vi "Offset Inline Buffers.vi"(8 "error in (no error)":errorcluster, 11 "Framework in":refnum<class "Framework.lvclass">) -> (0 "error out":errorcluster, 3 "Framework out":refnum<class "Framework.lvclass">)   [LabVIEW 2017, in "DSF Core.lvlib" / "Framework.lvclass"]
uses:
  Framework.lvclass
  Framework.lvclass/Framework.ctl
  Plugin/Plugin.lvclass
  Buffers/Buffers.lvclass
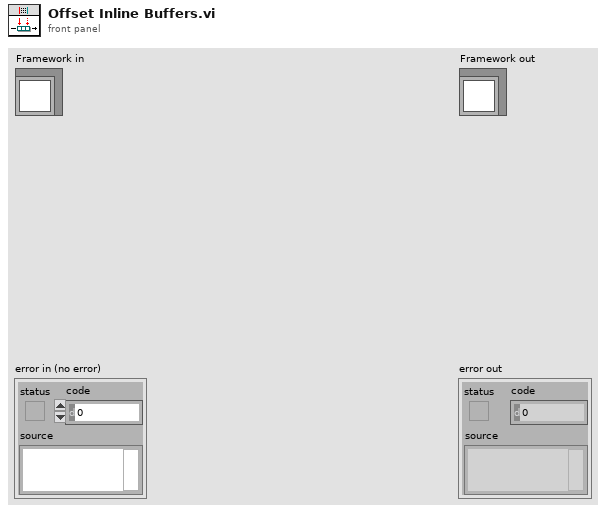
[diagram p1: front panel]
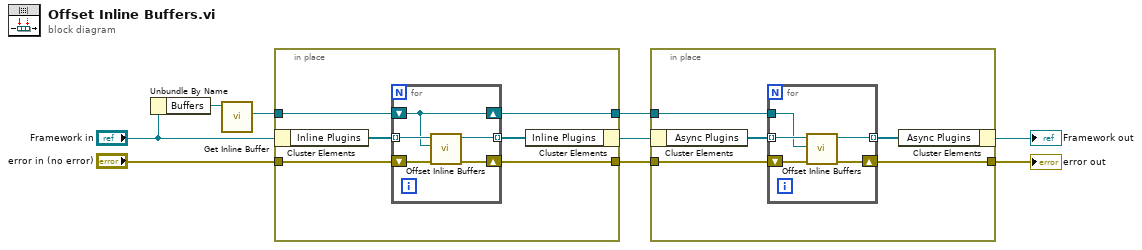
[diagram p0: block diagram]
diagram:
  n1 = Unbundle By Name("Framework in") -> ("Buffers"=w5:refnum<class "Buffers.lvclass">)
  n2 = call "Get Inline Buffer.vi"("Buffers in"=w5) -> ("Inline Buffer"=w1:refnum<class "Buffer.lvclass">)  [unwired: 9 in, 1 out]
  n3 = in-place {
    in-place-border: "error in (no error)" -> [w12]
    in-place-border: [w13] -> w8
    in-place-border: w1 -> [w11]
    in-place-border: [w10] -> w2
    n4 = in-place-cluster #1("Framework in") -> ("Inline Plugins"=w15:refnum<class "Plugin.lvclass">[])
    n5 = for {
      tunnel: w15 -> [w20] mode=indexing
      tunnel: [w19] -> w14 mode=indexing
      shift-right: [w18] -> w13
      shift-left: w12 -> [w17]
      shift-right: [w16] -> w10
      shift-left: w11 -> [w16]
      n6 = call "Offset Inline Buffers.vi"("error in (no error)"=w17, "Framework Inline Buffer"=w16, "Plugin in"=w20) -> ("error out"=w18:errorcluster, "Plugin out"=w19:refnum<class "Plugin.lvclass">)  [unwired: 7 in]
    }
    n7 = in-place-cluster #1("Inline Plugins"=w14) -> (w3:refnum<class "Framework.lvclass">)
  }
  n8 = in-place {
    in-place-border: w8 -> [w22]
    in-place-border: [w23] -> w6
    in-place-border: w2 -> [w21]
    n9 = in-place-cluster #2(w3) -> ("Async Plugins"=w25:refnum<class "Plugin.lvclass">[])
    n10 = for {
      tunnel: w25 -> [w30] mode=indexing
      tunnel: [w29] -> w24 mode=indexing
      shift-right: [w28] -> w23
      shift-left: w22 -> [w27]
      tunnel: w21 -> [w26]
      n11 = call "Offset Inline Buffers.vi"("error in (no error)"=w27, "Framework Inline Buffer"=w26, "Plugin in"=w30) -> ("error out"=w28:errorcluster, "Plugin out"=w29:refnum<class "Plugin.lvclass">)  [unwired: 7 in]
    }
    n12 = in-place-cluster #2("Async Plugins"=w24) -> (→"Framework out":refnum<class "Framework.lvclass">)
  }
  "error out" <- w6
